vi "Get Offset.vi"(8 "error in (no error)":errorcluster caption="错误输入（无错误）", 11 "Gif Image输入":refnum<class "Gif Image.lvclass">) -> (0 "error out":errorcluster caption="错误输出", 2 "Offset":i32, 3 "Gif Image输出":refnum<class "Gif Image.lvclass">)   [LabVIEW 2011, in "Gif Image.lvclass"]
uses:
  Gif Image.lvclass
  Gif Image.lvclass/Gif Image.ctl
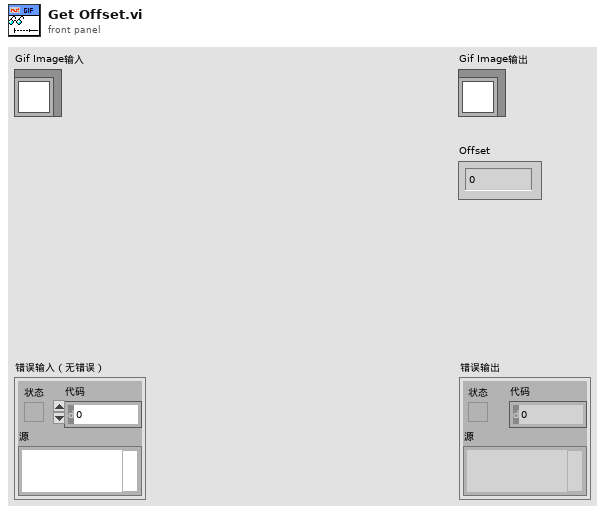
[diagram p1: front panel]
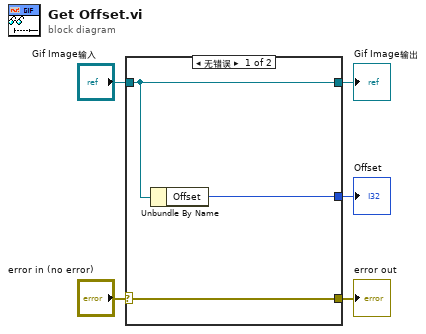
[diagram p0: block diagram]
diagram:
  n1 = case shown="无错误" "error in (no error)" {
    selector: "error in (no error)" -> [w8 w9]
    tunnel: [w8 w9] -> w4
    tunnel: [w7 w10] -> w2
    tunnel: "Gif Image输入" -> [w7 w10]
    tunnel: [w6 _] -> w1
    frame No Error {
      n2 = Unbundle By Name(w7) -> ("Offset"=w6:i32)
    }
    frame Error {
    }
  }
  "error out" <- w4
  "Gif Image输出" <- w2
  "Offset" <- w1
